vi "Event Receive.vi"(11 "Event Actor in":refnum<class "Event Actor.lvclass">) -> (2 "Event Msg":refnum<user-event>, 3 "Event Actor out":refnum<class "Event Actor.lvclass">)   [LabVIEW 2021, in "Event Actor.lvclass"]
uses:
  Event Actor.lvclass
  Msg/Msg.lvclass
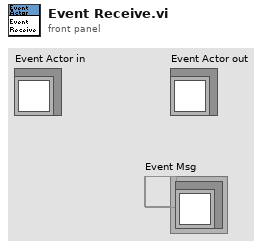
[diagram p1: front panel]
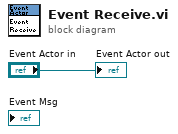
[diagram p0: block diagram]
diagram:
  "Event Actor out" <- "Event Actor in"
